vi "AJUSTE V-DIV.vi"(11 "y 2":dbl) -> (3 "y":dbl)   [LabVIEW 2019]
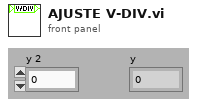
[diagram p1: front panel]
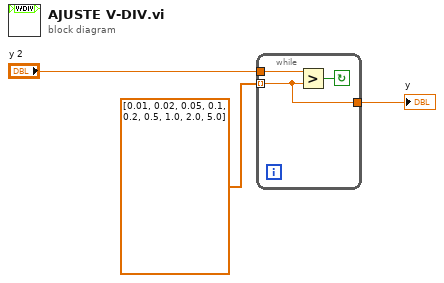
[diagram p0: block diagram]
diagram:
  n1 = while {
    tunnel: dbl[] [0.01, 0.02, 0.05, 0.1, 0.2, 0.5, 1.0, 2.0, 5.0] -> [w5] mode=indexing
    tunnel: "y 2" -> [w6]
    tunnel: [w5] -> w3
    stop <- w4 continue-if-true
    n2 = Greater?(x=w6, y=w5) -> (0:w4:bool)
  }
  "y" <- w3
